vi "Get Target Type.vi"(8 "error in (no error)":errorcluster, 11 "node ref in":T1) -> (0 "error out":errorcluster, 2 "Target Type":T2, 3 "node ref out":T1)   [LabVIEW 2014, in "SQLite editor node.lvclass"]
uses:
  SQLite editor node.lvclass
  <vilib>/NI/Tag Bus Module Framework/root configuration/Target Types.ctl
  <vilib>/NI/Configuration Framework/Node/NodeRef.ctl
  <vilib>/NI/Configuration Framework/Node/NISE_CEF_Node.lvclass
  <vilib>/NI/DCAF/Tag Editor Core/Configuration Editor/Classes/Targets/Targets.lvclass
  <vilib>/NI/DCAF/Tag Editor Core/Framework Configuration Classes/target configuration/PL_Target Configuration.lvclass/PL_Target Configuration.ctl
  <vilib>/NI/Configuration Framework/Node/NISE_CEF_Node.lvclass/NISE_CEF_Node.ctl
  <vilib>/NI/Configuration Framework/Node/ReadParent.vi
  <vilib>/NI/DCAF/Tag Editor Core/Framework Configuration Classes/target configuration/PL_Target Configuration.lvclass
  <vilib>/NI/Tag Bus Module Framework/root configuration/TBM configuration.lvclass
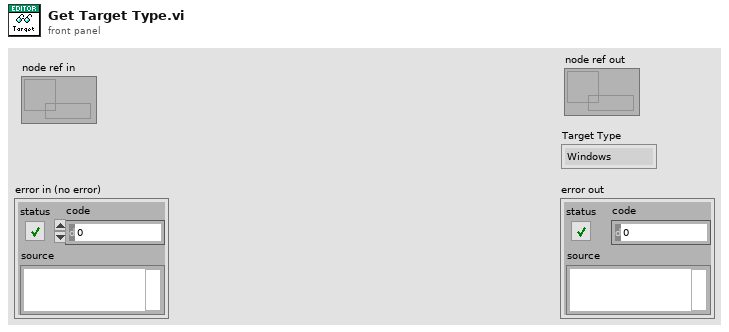
[diagram p1: front panel]
types:
  T1 = typedef "NISE_CEF_Node.lvclass/NodeRef.ctl" = refnum<data-value>
  T2 = typedef "TBM configuration.lvclass/Target Types.ctl" = enum16{"Windows", "Mac", "Linux", "Linux RT ARM", "VxWorks", "Pharlap", "Other", "Linux RT x64"}
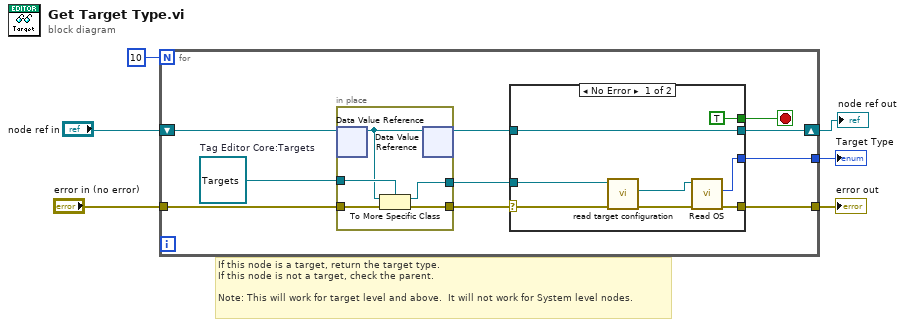
[diagram p0: block diagram]
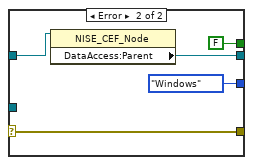
[diagram p2: hidden frame]
diagram:
  # "If this node is a target, return the target type.\nIf this node is not a target, check the parent.\n\nNote: This will work for target level and above.  It will not work for System level nodes."
  n1 = for {
    N: 10 -> [_]
    tunnel: [w11] -> w6
    shift-right: [w9] -> w1
    shift-left: "node ref in" -> [w16]
    tunnel: "error in (no error)" -> [w8]
    tunnel: [w7] -> w3
    stop <- w13 stop-if-true
    w15 = refnum<class "Targets.lvclass"> refnum  # Tag Editor Core:Targets
    n2 = in-place {
      in-place-border: w15 -> [w34]
      in-place-border: [w33] -> w12
      in-place-border: [w32] -> w14
      in-place-border: w8 -> [w30]
      n3 = in-place-dvr #1(w16) -> (w31:refnum<class "NISE_CEF_Node.lvclass">)  [unwired: 1 out]
      n4 = To More Specific Class(target class=w34, reference=w31, error in=w30) -> (specific class reference=w33:refnum<class "Targets.lvclass">, error out=w32:errorcluster)
      n5 = in-place-dvr #1(w31) -> (w10:T1)  [unwired: 1 out]
    }
    n6 = case shown="No Error" w14 {
      selector: w14 -> [w21 w25]
      tunnel: [TRUE FALSE] -> w13
      tunnel: w12 -> [w20 _]
      tunnel: [w19 Target_Types."Windows" ("Target Types")] -> w11
      tunnel: w10 -> [w18 w27]
      tunnel: [w18 w26] -> w9
      tunnel: [w17 w25] -> w7
      frame No Error {
        n7 = call <vilib>:"read target configuration.vi"("error in"=w21, "Targets in"=w20) -> ("error out"=w23:errorcluster, "Target Configuration"=w24:refnum<class "PL_Target Configuration.lvclass">)  [unwired: 7 in, 1 out]
        n8 = call <vilib>:"Read OS.vi"("error in"=w23, "PL_Target Configuration in"=w24) -> ("error out"=w17:errorcluster, "Target Types"=w19:T2)  [unwired: 7 in, 1 out]
      }
      frame Error {
        n9 = property class="NISE_CEF_Node"(reference=w27) -> ("DataAccess:Parent"=w26:T1)  [unwired: 1 in, 2 out]
      }
    }
  }
  "Target Type" <- w6
  "error out" <- w3
  "node ref out" <- w1
